vi "002 noms i cognoms.vi"() -> ()   [LabVIEW 2019]
panel:
  in  "stop":bool
  out "Format Into String":string
  in  "Cognoms":string
  in  "Nom":string
  out "Concatenated string":string
  in  "Cognoms":string
  in  "Nom":string
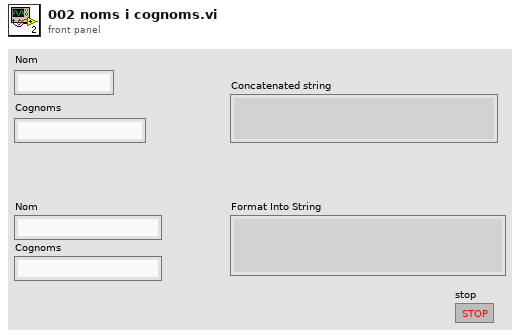
[diagram p1: front panel]
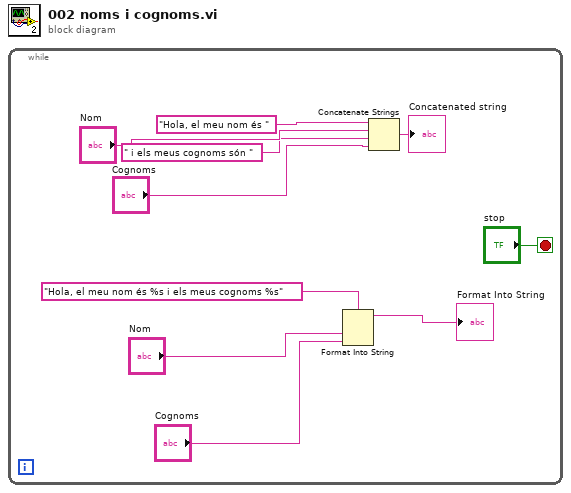
[diagram p0: block diagram]
diagram:
  n1 = while {
    stop <- "stop" stop-if-true
    n2 = Format Into String "Format Into String"(format string="Hola, el meu nom és %s i els meus cognoms %s" ("initial string"), "Nom", "Cognoms") -> (resulting string=→"Format Into String":string)  [unwired: 2 in, 1 out]
    n3 = Concatenate Strings("Hola, el meu nom és " ("string"), "Nom", " i els meus cognoms són " ("string"), "Cognoms") -> (→"Concatenated string":string)
  }
